vi "Set Slide SIze.vi"(6 "DPI":dbl=72.0, 8 "error in (no error)":errorcluster, 9 "Slide size":T1, 10 "File refnum":refnum<k7>) -> (0 "error out":errorcluster, 2 "File refnum out":refnum<k7>)   [LabVIEW 2020, in "lvpptx.lvlib"]
uses:
  lvpptx.lvlib
panel:
  # "Set slide size"
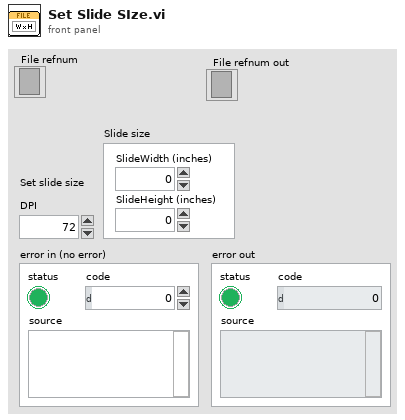
[diagram p1: front panel]
types:
  T1 = cluster{"SlideWidth (inches)":sgl, "SlideHeight (inches)":sgl}
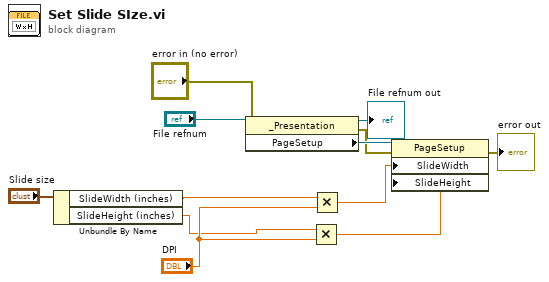
[diagram p0: block diagram]
diagram:
  n1 = Unbundle By Name("Slide size") -> ("SlideWidth (inches)"=w2:sgl, "SlideHeight (inches)"=w1:sgl)
  n2 = property class="_Presentation"(reference="File refnum", error in="error in (no error)") -> (reference out=→"File refnum out":refnum<k7>, error out=w7:errorcluster, "PageSetup"=w10:refnum<k7>)
  n3 = Multiply(x=w1, y="DPI") -> (x*y=w8:dbl)
  n4 = Multiply(x=w2, y="DPI") -> (x*y=w9:dbl)
  n5 = property class="PageSetup"(reference=w10, error in=w7, "SlideWidth"=w9, "SlideHeight"=w8) -> (error out=→"error out":errorcluster)  [unwired: 1 out]
